vi "OCT Processing OpenCL.vi"(0 "Data Format":T3, 1 "State":T4, 5 "Linear?":bool, 9 "Input Parameters":T2={"Points Per A-Scan"=0, "A-Scans per B-Scan"=0, "Voltage Range"=4.0, "Card Resolution (bits)"=16}, 11 "error in (no error)":errorcluster, 12 "Background":i32[](array[numeric]), 13 "Resample Array":i32[](array[numeric])) -> (3 "Time Out":bool, 4 "Processed OCT Data":T1, 10 "queue out":refnum<queue>, 14 "# elements in queue":i32, 15 "error out":errorcluster)   [LabVIEW 2014]
doc: "Functional global for processing OCT data. The data can either be 1 channel, 2 channel interleaved (ex. ATS 9462), or 2 channels appended (ATS 660). The output cluster Channel A and Channel B may be a single B-Scan or multople B-Scan stored in an array cluster. Same for the Raw Data Channel A and B."
uses:
  Type Defs/OCT Imaging Parameters Cluster.ctl
  OpenCL States.ctl
  Signal Processing/processing_states.ctl
  Type Defs/OCT DAQ Channel Data Type.ctl
  Type Defs/Processed OCT Data.ctl
panel:
  out "x-y":u32
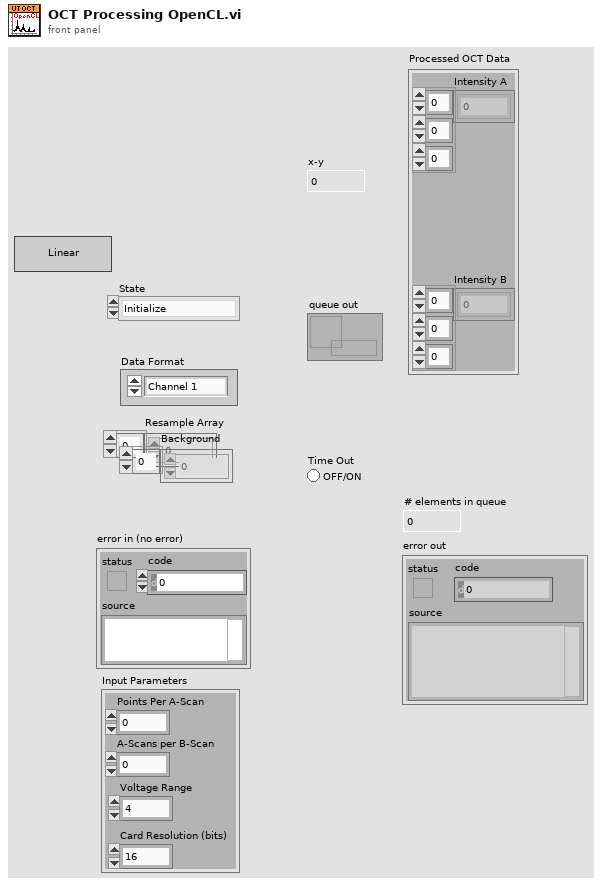
[diagram p1: front panel]
types:
  T1 = typedef "Processed OCT Data.ctl" = cluster{"Intensity A":sgl[][][], "Intensity B":sgl[][][]}
  T2 = typedef "OCT Imaging Parameters Cluster.ctl" = cluster{"Points Per A-Scan":i32, "A-Scans per B-Scan":i32, "Voltage Range":sgl, "Card Resolution (bits)":u16}
  T3 = typedef "OCT DAQ Channel Data Type.ctl" = enum16{"Channel 1", "Channel 2", "Channel 1 and 2"}
  T4 = typedef "processing_states.ctl" = enum16{"Initialize", "Set Background", "Update Imaging Parameters", "Get Queue", "Process Data", "Get Size", "Flush Data", "Set Reample Array", "Get Last Processed BScan", "Shutdown"}
  T5 = typedef "OpenCL States.ctl" = enum16{"Allocate Memory", "Get U16 Memory Dimension", "Compile Kernels", "Create Device", "Write", "Read", "Operate", "Delete Memory", "Delete"}
  T6 = cluster{"Magnitude":sgl[][][], "Phase":sgl[][][]}
  T7 = cluster{"Int B-Scan Channel A":sgl[][][], "Int B-Scan Channel B":sgl[][][]}
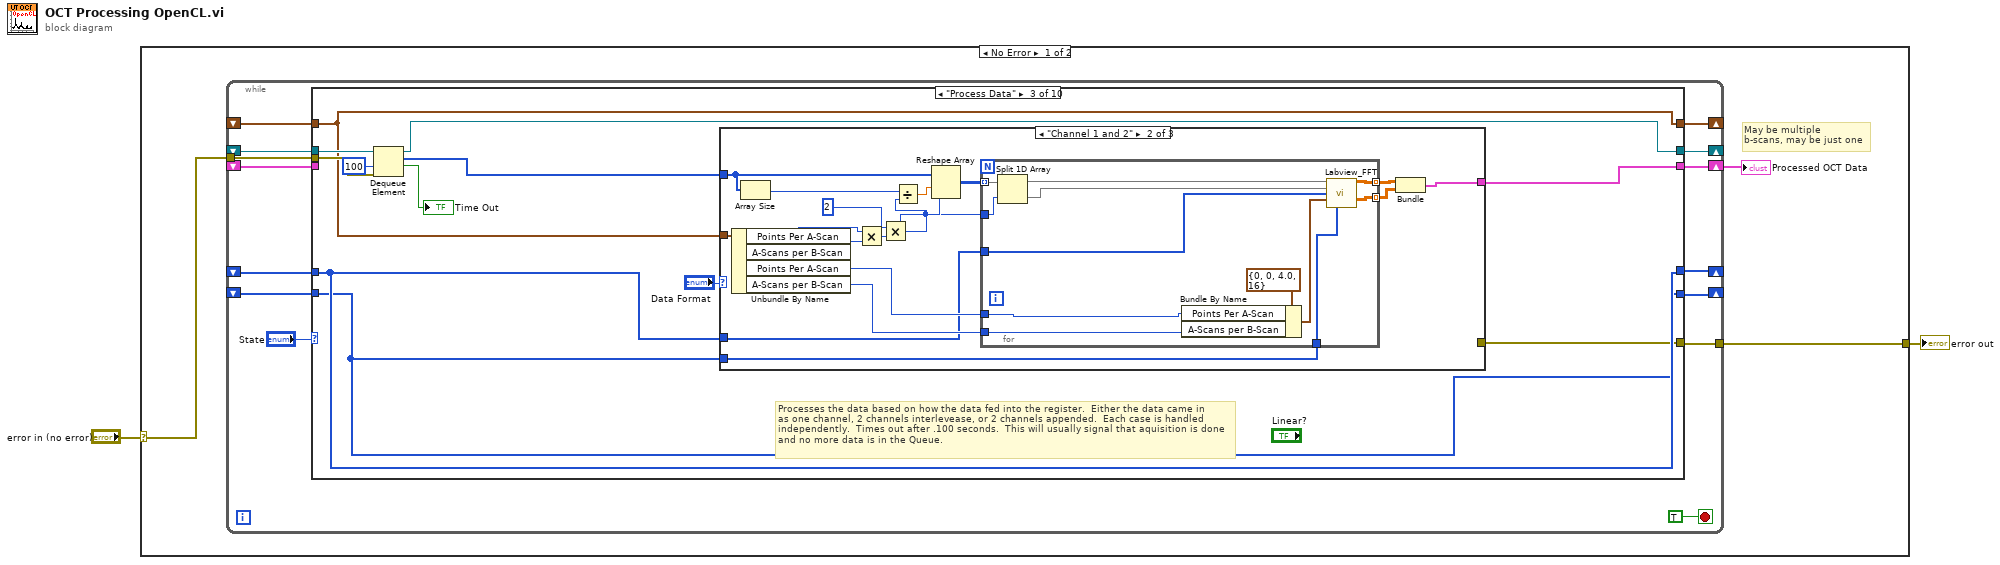
[diagram p0: block diagram]
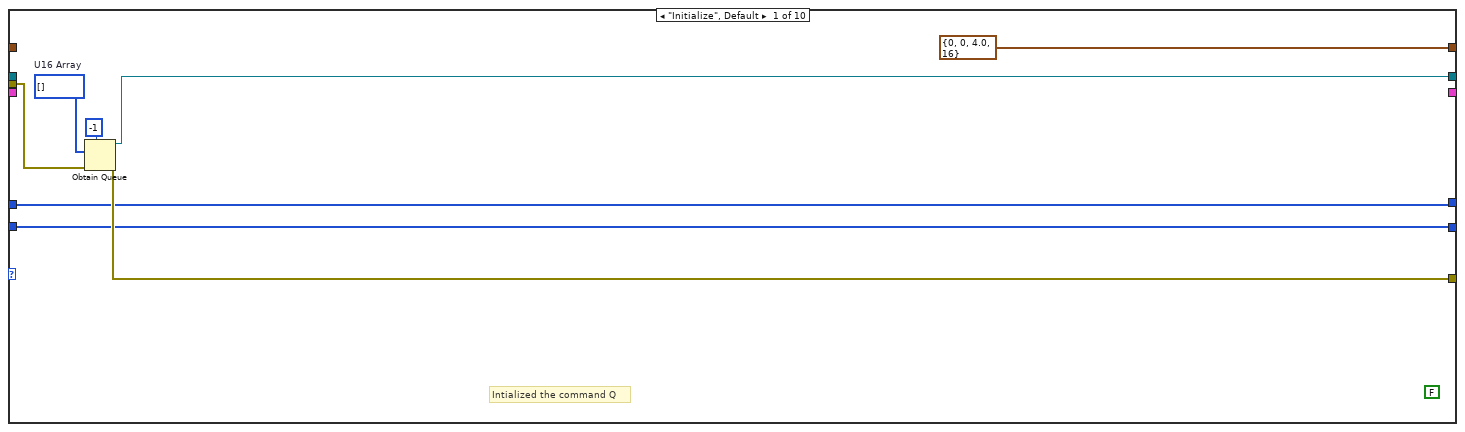
[diagram p2: hidden frame]
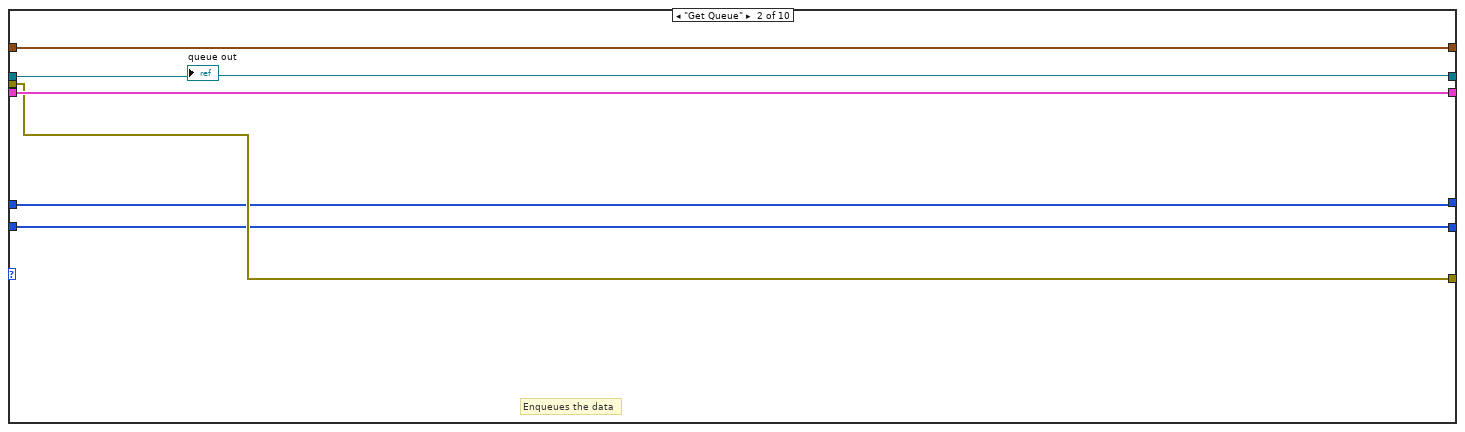
[diagram p3: hidden frame]
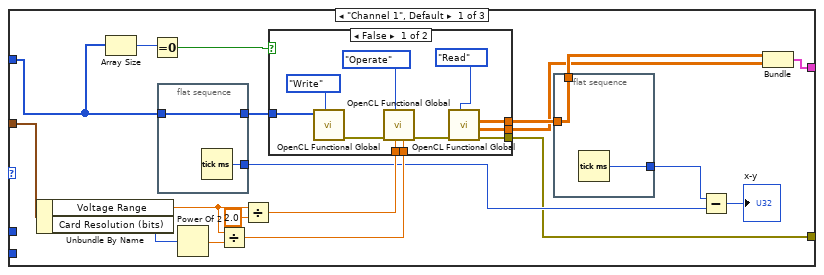
[diagram p4: hidden frame]
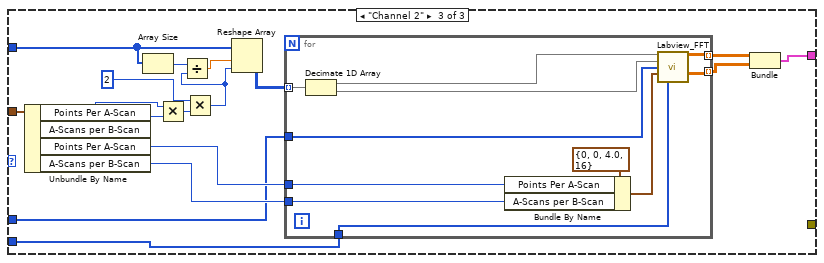
[diagram p6: hidden frame]
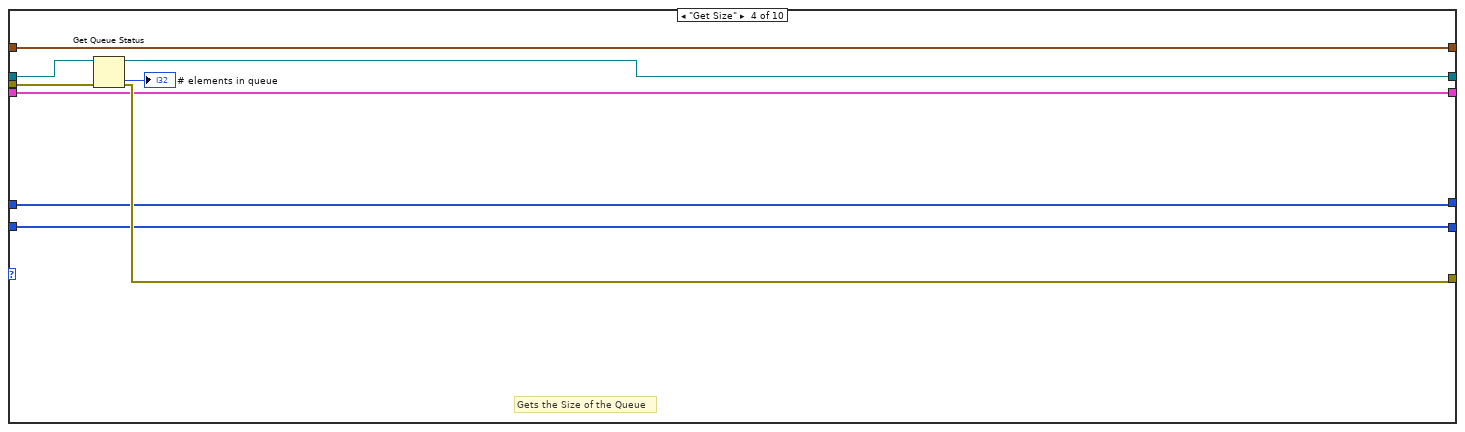
[diagram p7: hidden frame]
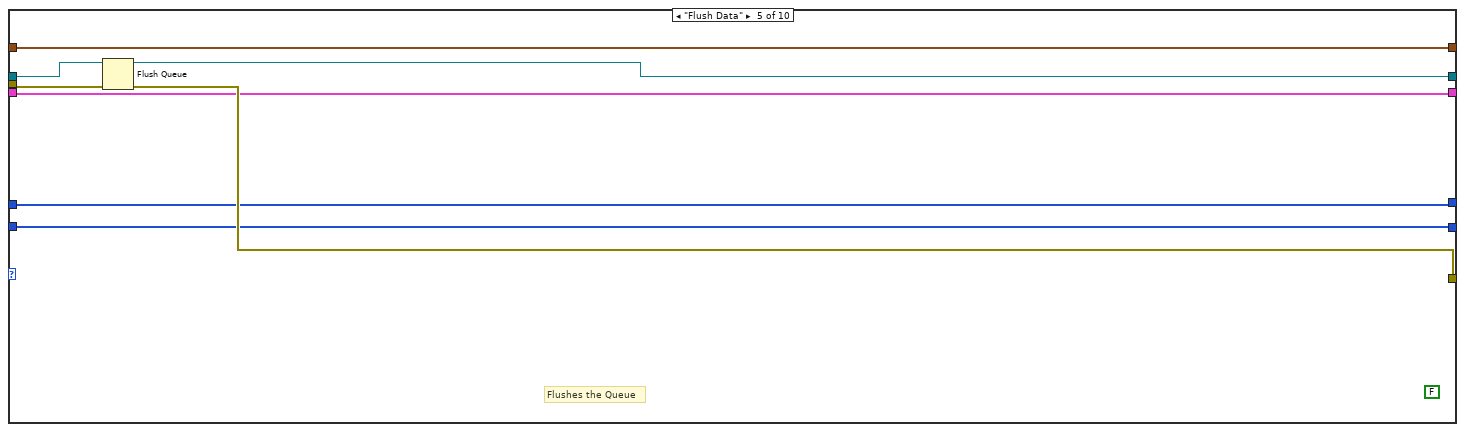
[diagram p8: hidden frame]
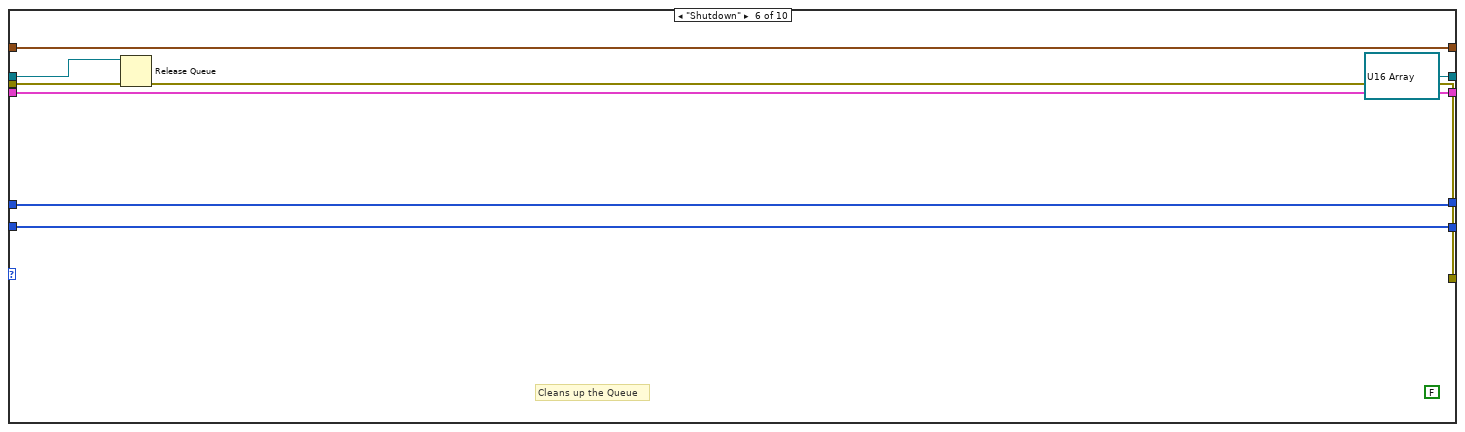
[diagram p9: hidden frame]
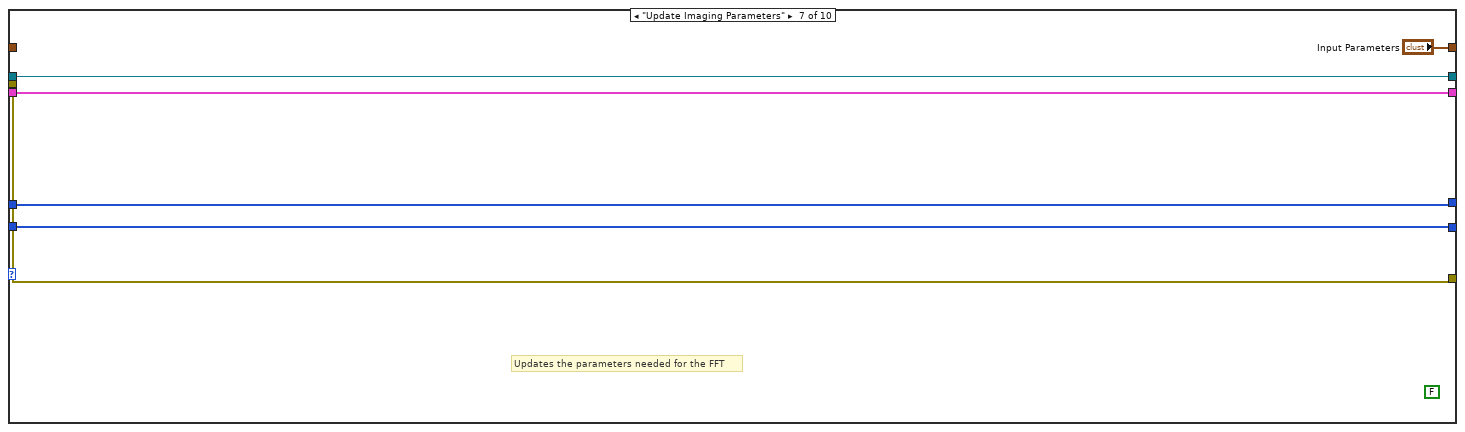
[diagram p10: hidden frame]
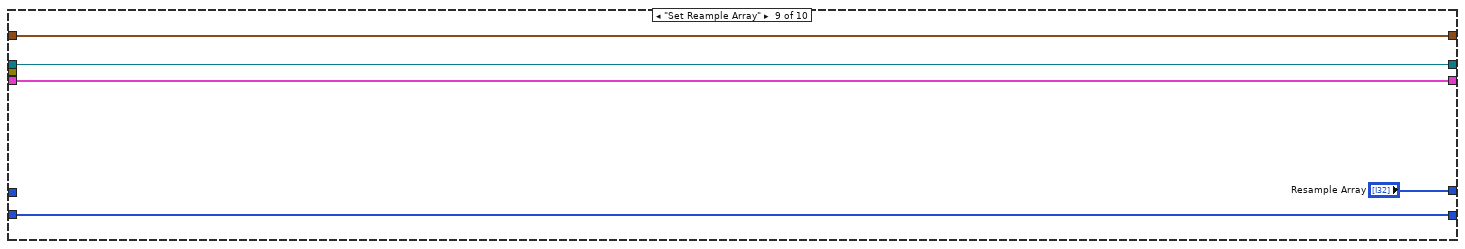
[diagram p12: hidden frame]
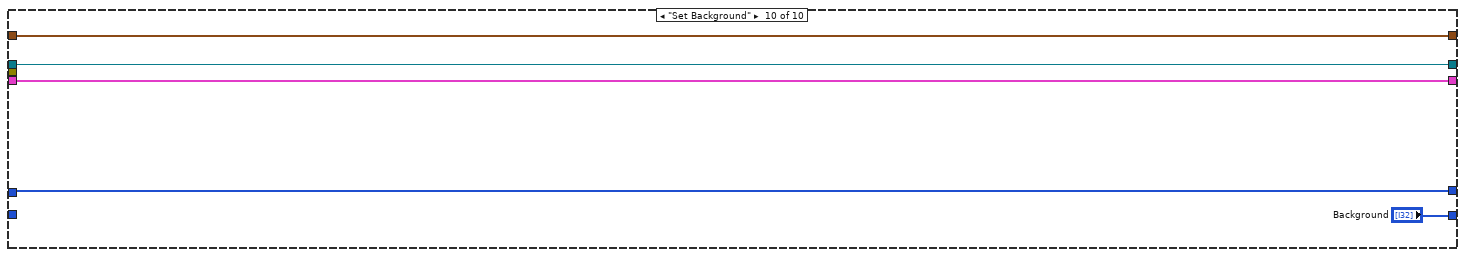
[diagram p13: hidden frame]
diagram:
  n1 = case shown="No Error" "error in (no error)" {
    selector: "error in (no error)" -> [w5 w183]
    tunnel: [w4 w183] -> w1
    frame No Error {
      # "May be multiple\nb-scans, may be just one"
      n2 = while {
        shift-right: [w12] -> _
        shift-left: _ -> [w17]
        tunnel: w5 -> [w18]
        tunnel: [w16] -> w4
        shift-right: [w15] -> _
        shift-left: _ -> [w13]
        shift-right: [w11] -> w3
        shift-left: _ -> [w10]
        shift-right: [w9] -> _
        shift-left: _ -> [w8]
        shift-right: [w6] -> _
        shift-left: _ -> [w7]
        stop <- TRUE stop-if-true
        n3 = case shown="\"Process Data\"" "State" {
          tunnel: [w26 w30 w44 w141 w150 refnum<queue> refnum ("queue out") w167 w172 w174 w180] -> w12
          tunnel: w18 -> [w27 w31 w43 w144 w152 w159 w166 _ _ _]
          tunnel: w17 -> [_ w30 w45 w145 w153 w161 w167 w172 w174 w180]
          tunnel: [w25 w31 w34 w142 w151 w158 w166 _ _ _] -> w16
          tunnel: [T2 {"Points Per A-Scan"=0, "A-Scans per B-Scan"=0, "Voltage Range"=4.0, "Card Resolution (bits)"=16} ("Input Parameters") w33 w42 w140 w149 w160 "Input Parameters" w171 w175 w181] -> w15
          tunnel: w13 -> [_ w33 w42 w140 w149 w160 _ w171 w175 w181]
          tunnel: [_ w32 w41 w139 w148 w157 w165 w170 w177 w182] -> w11
          tunnel: w10 -> [_ w32 _ w139 w148 w157 w165 w170 w177 w182]
          tunnel: [w21 w29 w36 w138 w147 w155 w163 w169 "Resample Array" w179] -> w9
          tunnel: w8 -> [w21 w29 w36 w138 w147 w155 w163 w169 _ w179]
          tunnel: w7 -> [w20 w28 w35 w137 w146 w154 w162 w168 w173 _]
          tunnel: [w20 w28 w35 w137 w146 w154 w162 w168 w173 "Background"] -> w6
          frame "Initialize", Default {
            w22 = u16[] []  # U16 Array
            (unwired) FALSE ("timed out?")
            # "Intialized the command Q"
            n4 = Obtain Queue(max queue size (-1, unlimited)=-1, element data type=w22, error in (no error)=w27) -> (queue out=w26:refnum<queue>, error out=w25:errorcluster)  [unwired: 2 in, 1 out]
          }
          frame "Get Queue" {
            # "Enqueues the data"
            "queue out" <- w30
          }
          frame "Process Data" {
            # "Processes the data based on how the data fed into the register.  Either the data came in\nas one channel, 2 channels interlevease, or 2 channels appended.  Each case is handled\nindependently.  Times out after .100 seconds.  This will usually signal that aquisition is done\nand no more data is in the Queue."
            n5 = Dequeue Element(queue=w45, timeout in ms (-1)=100, error in (no error)=w43) -> (queue out=w44:refnum<queue>, element=w37:u16[], timed out?=→"Time Out":bool)  [unwired: 1 out]
            n6 = case shown="\"Channel 1 and 2\"" "Data Format" {
              tunnel: w37 -> [w46 w94 w123]
              tunnel: w42 -> [w64 w95 w124]
              tunnel: [w50 w89 w109] -> w41
              tunnel: w36 -> [_ w82 w112]
              tunnel: w35 -> [_ w81 w111]
              tunnel: [w49 _ _] -> w34
              frame "Channel 1", Default {
                n7 = Unbundle By Name(w64) -> ("Voltage Range"=w59:sgl, "Card Resolution (bits)"=w61:u16)
                n8 = Array Size(array=w46) -> (size(s)=w48:i32)
                n9 = Equal To 0?(x=w48) -> (x = 0?=w47:bool)
                n10 = flat-sequence {
                  tunnel: [w79] -> w57
                  tunnel: w46 -> [w79]
                  tunnel: [w78] -> w52
                  frame #0 {
                    n11 = Tick Count (ms)() -> (millisecond timer value=w78:u32)
                  }
                }
                n12 = Power Of 2(x=w61) -> (2^x=w60:dbl)
                n13 = Divide(x=w59, y=w60) -> (x/y=w58:dbl)
                n14 = Divide(x=w59, y=sgl 2.0) -> (x/y=w63:sgl)
                n15 = case shown="False" w47 {
                  tunnel: w63 -> [w75 _]
                  tunnel: w58 -> [w74 _]
                  tunnel: w57 -> [w68 _]
                  tunnel: [w67 _] -> w55
                  tunnel: [w66 _] -> w54
                  tunnel: [w65 _] -> w49
                  frame False {
                    n16 = call "OpenCL Functional Global.vi"("States"=OpenCL_States."Write", "B-Scan"=w68) -> ("Error Out"=w71:errorcluster)  [unwired: 6 in, 3 out]
                    n17 = call "OpenCL Functional Global.vi"("Gain"=w74, "Bias"=w75, "States"=OpenCL_States."Operate", "Error In"=w71) -> ("Error Out"=w70:errorcluster)  [unwired: 4 in, 3 out]
                    n18 = call "OpenCL Functional Global.vi"("States"=OpenCL_States."Read", "Error In"=w70) -> ("Error Out"=w65:errorcluster, "Phase"=w66:sgl[][][], "Magnitude"=w67:sgl[][][])  [unwired: 6 in, 1 out]
                  }
                  frame True {
                  }
                }
                n19 = flat-sequence {
                  tunnel: [w77] -> w56
                  tunnel: w55 -> [w77]
                  tunnel: [w76] -> w53
                  frame #0 {
                    n20 = Tick Count (ms)() -> (millisecond timer value=w76:u32)
                  }
                }
                n21 = Subtract(x=w53, y=w52) -> (x-y=→"x-y":u32)
                n22 = Bundle("Magnitude"=w56, "Phase"=w54) -> (w50:T6)  [unwired: 1 in]
              }
              frame "Channel 1 and 2" {
                n23 = Unbundle By Name(w95) -> ("Points Per A-Scan"=w88:i32, "A-Scans per B-Scan"=w87:i32, "Points Per A-Scan"=w92:i32, "A-Scans per B-Scan"=w91:i32)
                n24 = Array Size(array=w94) -> (size(s)=w96:i32)
                n25 = Multiply(x=w88, y=w87) -> (x*y=w83:i32)
                n26 = Multiply(x=2 ("y"), y=w83) -> (x*y=w84:i32)
                n27 = Divide(x=w96, y=w84) -> (x/y=w85:dbl)
                n28 = Reshape Array(w94, w85, w84) -> (w93:u16[][])
                n29 = for {
                  tunnel: w93 -> [w108] mode=indexing
                  tunnel: w92 -> [w101]
                  tunnel: w91 -> [w105]
                  tunnel: [w104] -> w90 mode=indexing
                  tunnel: [w103] -> w80 mode=indexing
                  tunnel: w83 -> [w102]
                  tunnel: w82 -> [w98]
                  tunnel: w81 -> [w97]
                  n30 = Split 1D Array(array=w108, index=w102) -> (first subarray=w100:u16[], second subarray=w99:u16[])
                  n31 = Bundle By Name(cluster=T2 {"Points Per A-Scan"=0, "A-Scans per B-Scan"=0, "Voltage Range"=4.0, "Card Resolution (bits)"=16} ("input cluster"), "Points Per A-Scan"=w101, "A-Scans per B-Scan"=w105) -> (w106:T2)
                  n32 = call "Labview_FFT.vi"("Channel A"=w100, "Channel B"=w99, "Resample Array"=w98, "Input Parameters"=w106, "Background"=w97) -> ("Int B-Scan Channel A"=w104:sgl[][], "Int B-Scan Channel B"=w103:sgl[][])  [unwired: 9 in]
                }
                n33 = Bundle("Int B-Scan Channel A"=w90, "Int B-Scan Channel B"=w80) -> (w89:T7)  [unwired: 1 in]
              }
              frame "Channel 2" {
                n34 = Unbundle By Name(w124) -> ("Points Per A-Scan"=w118:i32, "A-Scans per B-Scan"=w117:i32, "Points Per A-Scan"=w121:i32, "A-Scans per B-Scan"=w120:i32)
                n35 = Array Size(array=w123) -> (size(s)=w125:i32)
                n36 = Multiply(x=w118, y=w117) -> (x*y=w116:i32)
                n37 = Multiply(x=2, y=w116) -> (x*y=w113:i32)
                n38 = Divide(x=w125, y=w113) -> (x/y=w114:dbl)
                n39 = Reshape Array(w123, w114, w113) -> (w122:u16[][])
                n40 = for {
                  tunnel: w122 -> [w136] mode=indexing
                  tunnel: w121 -> [w130]
                  tunnel: w120 -> [w134]
                  tunnel: [w132] -> w119 mode=indexing
                  tunnel: [w131] -> w110 mode=indexing
                  tunnel: w112 -> [w127]
                  tunnel: w111 -> [w126]
                  n41 = Decimate 1D Array(w136) -> (w129:u16[], w128:u16[])
                  n42 = Bundle By Name(cluster=T2 {"Points Per A-Scan"=0, "A-Scans per B-Scan"=0, "Voltage Range"=4.0, "Card Resolution (bits)"=16} ("input cluster"), "Points Per A-Scan"=w130, "A-Scans per B-Scan"=w134) -> (w133:T2)
                  n43 = call "Labview_FFT.vi"("Channel A"=w129, "Channel B"=w128, "Resample Array"=w127, "Input Parameters"=w133, "Background"=w126) -> ("Int B-Scan Channel A"=w132:sgl[][], "Int B-Scan Channel B"=w131:sgl[][])  [unwired: 9 in]
                }
                n44 = Bundle("Int B-Scan Channel A"=w119, "Int B-Scan Channel B"=w110) -> (w109:T7)  [unwired: 1 in]
              }
            }
          }
          frame "Get Size" {
            # "Gets the Size of the Queue"
            n45 = Get Queue Status(queue=w145, error in (no error)=w144) -> (queue out=w141:refnum<queue>, error out=w142:errorcluster, # elements in queue=→"# elements in queue":i32)  [unwired: 1 in, 5 out]
          }
          frame "Flush Data" {
            (unwired) FALSE ("timed out?")
            # "Flushes the Queue"
            n46 = Flush Queue(queue=w153, error in (no error)=w152) -> (queue out=w150:refnum<queue>, error out=w151:errorcluster)  [unwired: 1 out]
          }
          frame "Shutdown" {
            (unwired) FALSE ("timed out?")
            # "Cleans up the Queue"
            n47 = Release Queue(queue=w161, error in (no error)=w159) -> (error out=w158:errorcluster)  [unwired: 1 in, 2 out]
          }
          frame "Update Imaging Parameters" {
            (unwired) FALSE ("timed out?")
            # "Updates the parameters needed for the FFT"
          }
          frame "Get Last Processed BScan" {
            # "Just executes to get the last set of data from the shift register"
          }
          frame "Set Reample Array" {
          }
          frame "Set Background" {
          }
        }
      }
      "Processed OCT Data" <- w3
    }
    frame Error {
    }
  }
  "error out" <- w1
